vi "Wvfm5ToDbl5Avg.vi"(11 "Wvfm":dynamicdata(waveform)) -> (0 "Ch3Avg":dbl, 1 "Ch2Avg":dbl, 2 "Ch1Avg":dbl, 3 "Ch0Avg":dbl, 4 "Ch4Avg":dbl)   [LabVIEW 2017]
uses:
  <vilib>/Analysis/baseanly.llb/Mean (DBL).vi
  <vilib>/Waveform/WDTOps.llb/WDT Index Channel DBL.vi
  <vilib>/Analysis/NI_AALBase.lvlib
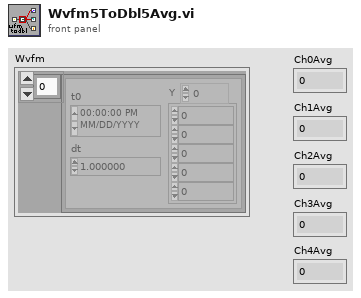
[diagram p1: front panel]
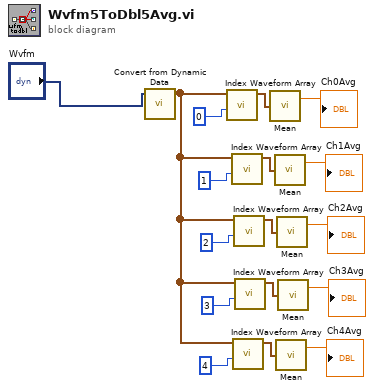
[diagram p0: block diagram]
diagram:
  n1 = call "Convert from Dynamic Data"("Dynamic Data Type"="Wvfm") -> ("Array of Waveform"=w17:waveform(dbl)[])  [unwired: 3 in]
  n2 = call-poly <vilib>:"Index Waveform Array.vi"("index"=0, "waveform array"=w17) -> ("waveform"=w3:waveform(dbl))  [unwired: 8 in, 1 out]
  n3 = call-poly <vilib>:"Index Waveform Array.vi"("index"=1, "waveform array"=w17) -> ("waveform"=w6:waveform(dbl))  [unwired: 8 in, 1 out]
  n4 = call-poly <vilib>:"Index Waveform Array.vi"("index"=4, "waveform array"=w17) -> ("waveform"=w15:waveform(dbl))  [unwired: 8 in, 1 out]
  n5 = call-poly <vilib>:"Index Waveform Array.vi"("index"=2, "waveform array"=w17) -> ("waveform"=w9:waveform(dbl))  [unwired: 8 in, 1 out]
  n6 = call-poly <vilib>:"Index Waveform Array.vi"("index"=3, "waveform array"=w17) -> ("waveform"=w12:waveform(dbl))  [unwired: 8 in, 1 out]
  n7 = call-poly <vilib>:"Mean.vi"("X"=w3) -> ("mean"=→"Ch0Avg":dbl)  [unwired: 1 out]
  n8 = call-poly <vilib>:"Mean.vi"("X"=w6) -> ("mean"=→"Ch1Avg":dbl)  [unwired: 1 out]
  n9 = call-poly <vilib>:"Mean.vi"("X"=w15) -> ("mean"=→"Ch4Avg":dbl)  [unwired: 1 out]
  n10 = call-poly <vilib>:"Mean.vi"("X"=w9) -> ("mean"=→"Ch2Avg":dbl)  [unwired: 1 out]
  n11 = call-poly <vilib>:"Mean.vi"("X"=w12) -> ("mean"=→"Ch3Avg":dbl)  [unwired: 1 out]
